vi "Result.Equipment List Item to 1D Array.vi"(9 "Eq Item":T1, 11 "Category":string) -> (3 "List":string[](array[string]))   [LabVIEW 2018]
uses:
  Result XML/TestResult.HW Item.ctl
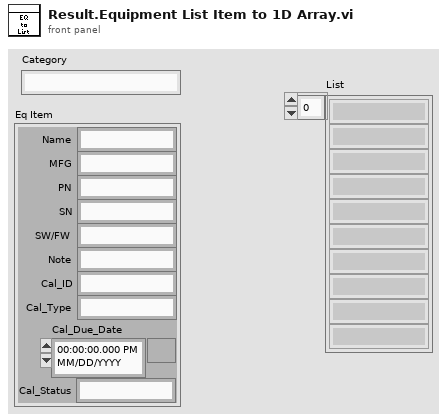
[diagram p1: front panel]
types:
  T1 = typedef "TestResult.HW Item.ctl" = cluster{"Name":string, "MFG":string, "PN":string, "SN":string, "SW/FW":string, "Note":string, "Cal_ID":string, "Cal_Type":string, "Cal_Due_Date":timestamp, "Cal_Status":string}
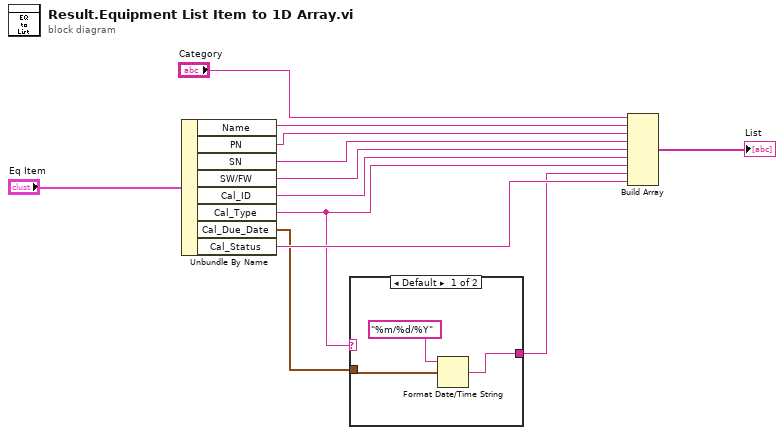
[diagram p0: block diagram]
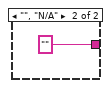
[diagram p2: hidden frame]
diagram:
  n1 = Unbundle By Name("Eq Item") -> ("Name"=w12:string, "PN"=w5:string, "SN"=w11:string, "SW/FW"=w10:string, "Cal_ID"=w9:string, "Cal_Type"=w3:string, "Cal_Due_Date"=w2:timestamp, "Cal_Status"=w8:string)
  n2 = case shown="Default" w3 {
    tunnel: w2 -> [w15 _]
    tunnel: [w13 ""] -> w1
    frame Default {
      n3 = Format Date/Time String(time format string (%c)="%m/%d/%Y", seconds (now)=w15) -> (date/time string=w13:string)  [unwired: 1 in]
    }
    frame "", "N/A" {
    }
  }
  n4 = Build Array("Category", w12, w5, w11, w10, w9, w3, w1, w8) -> (→"List":string[])
